vi "Example Local Queue Server-Client.vi"() -> ()   [LabVIEW 2013]
uses:
  MQTT_LocalQueue/Connection/LocalQueueConnection.lvclass
  <vilib>/LabVIEW Open Source Project/Connection/Connection/Connection.lvclass
panel:
  out "server connected":bool
  out "client connected":bool
  out "Comm OK":bool
  out "value":dbl
  out "listener error":errorcluster
  out "client session error":errorcluster
  out "server session error":errorcluster
  out "Bytes":u8[](array[numeric]) format="%08b"
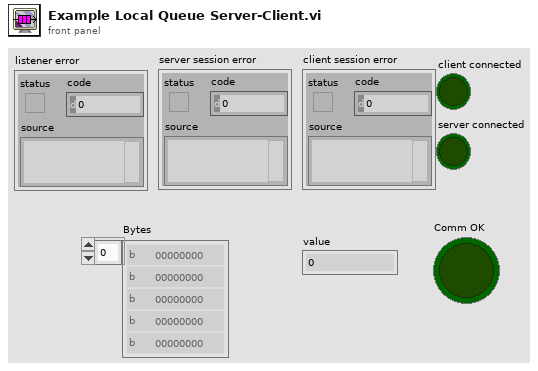
[diagram p1: front panel]
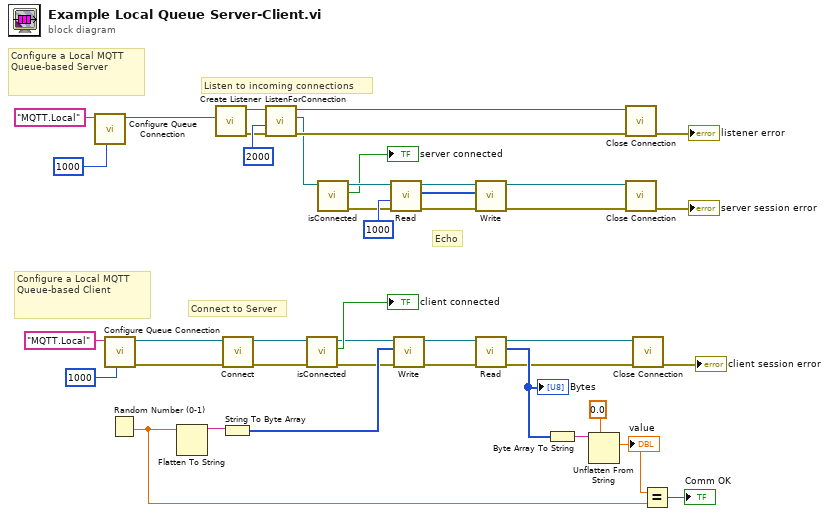
[diagram p0: block diagram]
diagram:
  # "Configure a Local MQTT Queue-based Client"
  # "Connect to Server"
  # "Echo"
  # "Listen to incoming connections"
  # "Configure a Local MQTT Queue-based Server"
  n1 = call "Configure Queue Connection.vi"("timeout (500 ms)"=1000 ("timeout (100ms)"), "Queue Name"="MQTT.Local") -> ("LocalQueueConnection"=w37:refnum<class "LocalQueueConnection.lvclass">)  [unwired: 8 in, 1 out]
  n2 = call "Configure Queue Connection.vi"("timeout (500 ms)"=1000 ("timeout (100ms)"), "Queue Name"="MQTT.Local") -> ("error out"=w28:errorcluster, "LocalQueueConnection"=w32:refnum<class "LocalQueueConnection.lvclass">)  [unwired: 8 in]
  n3 = Random Number (0-1)() -> (number: 0 to 1=w11:dbl)
  n4 = Flatten To String(anything=w11) -> (data string=w25:string)  [unwired: 3 in, 2 out]
  n5 = call <vilib>:"Create Listener.vi"("Connection Configuration"=w37) -> ("error out"=w38:errorcluster, "Listener"=w41:refnum<class "LocalQueueConnection.lvclass">)  [unwired: 9 in]
  n6 = String To Byte Array(string=w25) -> (unsigned byte array=w24:u8[])
  n7 = call <vilib>:"Connect.vi"("error in (no error)"=w28, "Connection in"=w32) -> ("error out"=w6:errorcluster, "Connection out"=w8:refnum<class "LocalQueueConnection.lvclass">)  [unwired: 8 in]
  n8 = call <vilib>:"ListenForConnection.vi"("error in (no error)"=w38, "timeout (2000 ms)"=2000 ("bytes to read (100)"), "Listener"=w41) -> ("error out"=w18:errorcluster, "Connection"=w4:refnum<class "Connection.lvclass">, "Listener out"=w39:refnum<class "LocalQueueConnection.lvclass">)  [unwired: 5 in, 1 out]
  n9 = call <vilib>:"isConnected.vi"("error in (no error)"=w6, "Connection in"=w8) -> ("error out"=w5:errorcluster, "connected"=→"client connected":bool, "Connection out"=w7:refnum<class "LocalQueueConnection.lvclass">)  [unwired: 7 in]
  n10 = call <vilib>:"isConnected.vi"("Connection in"=w4) -> ("error out"=w2:errorcluster, "connected"=→"server connected":bool, "Connection out"=w3:refnum<class "Connection.lvclass">)  [unwired: 8 in]
  n11 = call <vilib>:"Read.vi"("error in (no error)"=w2, "timeout (2000 ms)"=1000 ("bytes to read (100)"), "TCPConnection in"=w3) -> ("error out"=w30:errorcluster, "Bytes"=w34:u8[], "TCPConnection out"=w35:refnum<class "Connection.lvclass">)  [unwired: 4 in, 2 out]
  n12 = call <vilib>:"Write.vi"("error in (no error)"=w5, "Bytes"=w24, "Connection in"=w7) -> ("error out"=w29:errorcluster, "Connection"=w31:refnum<class "LocalQueueConnection.lvclass">)  [unwired: 7 in]
  n13 = call <vilib>:"Write.vi"("error in (no error)"=w30, "Bytes"=w34, "Connection in"=w35) -> ("error out"=w16:errorcluster, "Connection"=w26:refnum<class "Connection.lvclass">)  [unwired: 7 in]
  n14 = call <vilib>:"Read.vi"("error in (no error)"=w29, "TCPConnection in"=w31) -> ("error out"=w15:errorcluster, "Bytes"=w23:u8[], "TCPConnection out"=w13:refnum<class "LocalQueueConnection.lvclass">)  [unwired: 5 in, 2 out]
  "Bytes" <- w23
  n15 = Byte Array To String(unsigned byte array=w23) -> (string=w22:string)
  n16 = Unflatten From String(type=0.0, binary string=w22) -> (value=w12:dbl)  [unwired: 3 in, 2 out]
  "value" <- w12
  n17 = call <vilib>:"Close Connection.vi"("error in (no error)"=w18, "Connection in"=w39) -> ("error out"=→"listener error":errorcluster)  [unwired: 8 in, 1 out]
  n18 = call <vilib>:"Close Connection.vi"("error in (no error)"=w16, "Connection in"=w26) -> ("error out"=→"server session error":errorcluster)  [unwired: 8 in, 1 out]
  n19 = call <vilib>:"Close Connection.vi"("error in (no error)"=w15, "Connection in"=w13) -> ("error out"=→"client session error":errorcluster)  [unwired: 8 in, 1 out]
  n20 = Equal?(x=w12, y=w11) -> (x = y?=→"Comm OK":bool)
